vi "poly_ref_tools_eco_plus.vi"(4 "code (w/out eco)":i32) -> (1 "code (+ eco)":i32)   [LabVIEW 2015]
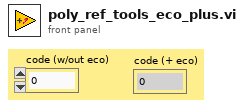
[diagram p1: front panel]
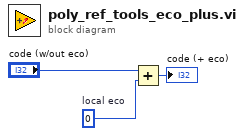
[diagram p0: block diagram]
diagram:
  w1 = 0  # local eco
  n1 = Add(x="code (w/out eco)", y=w1) -> (x+y=→"code (+ eco)":i32)
